vi "Get Datatype.vi"(11 "Value":variant) -> (3 "datatypes":T1)   [LabVIEW 2025, in "Tools.lvlib"]
uses:
  Tools/Tools.lvlib
  Tools/Datatypes.ctl
  <vilib>/Utility/Data Type/Type Definitions/Data Type.ctl
  <vilib>/Utility/Data Type/NI_Data Type.lvlib
panel:
  out "name":string
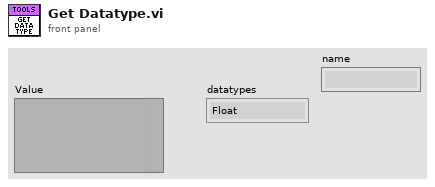
[diagram p1: front panel]
types:
  T1 = typedef "Tools.lvlib/Datatypes.ctl" = enum16{"Float", "Int", "String", "String Array", "Int Array", "Float Array", "Bool Array", "Bool", "Invalid"}
  T2 = typedef "NI_Data Type.lvlib/Data Type.ctl" = enum8{"Invalid Type", "Void", "I8", "I16", "I32", "I64", "U8", "U16", "U32", "U64", "Single Float", "Double Float", "Extended Float", "Single Complex", "Double Complex", "Extended Complex", "Enum U8", "Enum U16", "Enum U32", "Enum U64", "Single Float With Unit", "Double Float With Unit", "Extended Float With Unit", "Single Complex with Unit", "Double Complex with Unit", "Extended Complex with Unit", "Boolean", "String", "Path", "Picture", "Tag", "Array", "Cluster", "Variant", "LV Variant", "Waveform", "Timestamp", "Digital Waveform", "Digital Data", "ExpressData", "Refnum", "External Data", "VI", "Poly VI", "LabVIEW Class Instance", "Fixed Point", "Set Collection", "Map Collection"}
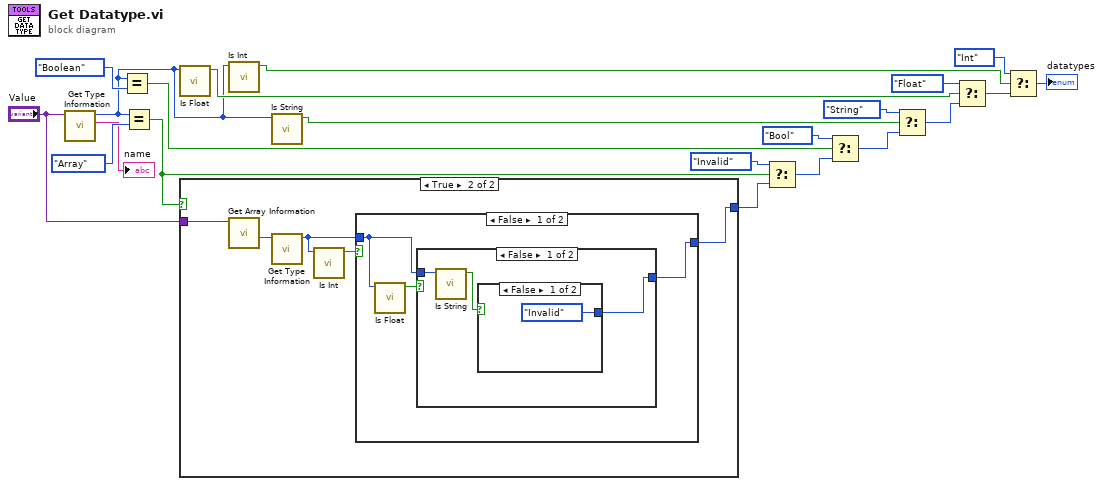
[diagram p0: block diagram]
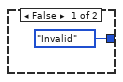
[diagram p2: hidden frame]
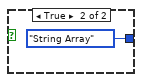
[diagram p3: hidden frame]
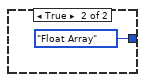
[diagram p4: hidden frame]
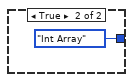
[diagram p5: hidden frame]
diagram:
  n1 = call <vilib>:"Get Type Information.vi"("variant"="Value") -> ("name"=→"name":string, "type"=w8:T2)  [unwired: 6 in, 3 out]
  n2 = Equal?(x=w8, y=Data_Type."Boolean" ("Type Enum")) -> (x = y?=w21:bool)
  n3 = Equal?(x=w8, y=Data_Type."Array" ("Type Enum")) -> (x = y?=w3:bool)
  n4 = call "Is Float.vi"("type"=w8) -> ("Boolean"=w14:bool)  [unwired: 10 in]
  n5 = case shown="True" w3 {
    tunnel: [Datatypes."Invalid" ("t") w27] -> w2
    tunnel: "Value" -> [_ w26]
    frame False {
    }
    frame True {
      n6 = call <vilib>:"Get Array Information.vi"("variant"=w26) -> ("array element data type"=w23:variant)  [unwired: 7 in, 3 out]
      n7 = call <vilib>:"Get Type Information.vi"("variant"=w23) -> ("type"=w24:T2)  [unwired: 6 in, 4 out]
      n8 = call "Is Int.vi"("type"=w24) -> ("is int?"=w25:bool)  [unwired: 10 in]
      n9 = case shown="False" w25 {
        tunnel: [w30 Datatypes."Int Array" ("t")] -> w27
        tunnel: w24 -> [w28 _]
        frame False {
          n10 = call "Is Float.vi"("type"=w28) -> ("Boolean"=w29:bool)  [unwired: 10 in]
          n11 = case shown="False" w29 {
            tunnel: [w33 Datatypes."Float Array" ("t")] -> w30
            tunnel: w28 -> [w32 _]
            frame False {
              n12 = call "Is String.vi"("type"=w32) -> ("Boolean"=w31:bool)  [unwired: 10 in]
              n13 = case shown="False" w31 {
                tunnel: [Datatypes."Invalid" ("t") Datatypes."String Array" ("t")] -> w33
                frame False {
                }
                frame True {
                }
              }
            }
            frame True {
            }
          }
        }
        frame True {
        }
      }
    }
  }
  n14 = call "Is Int.vi"("type"=w8) -> ("is int?"=w4:bool)  [unwired: 10 in]
  n15 = call "Is String.vi"("type"=w8) -> ("Boolean"=w15:bool)  [unwired: 10 in]
  n16 = Select(t=Datatypes."Invalid", s=w3, f=w2) -> (s? t:f=w7:T1)
  n17 = Select(t=Datatypes."Bool" ("f"), s=w21, f=w7) -> (s? t:f=w19:T1)
  n18 = Select(t=Datatypes."String", s=w15, f=w19) -> (s? t:f=w16:T1)
  n19 = Select(t=Datatypes."Float", s=w14, f=w16) -> (s? t:f=w12:T1)
  n20 = Select(t=Datatypes."Int", s=w4, f=w12) -> (s? t:f=→"datatypes":T1)
